vi "RGB2labMAT1.vi"(3 "sRL":dbl[](array[numeric]), 4 "sGL":dbl[](array[numeric]), 5 "sRL":dbl[](array[numeric])) -> (0 "b":dbl[](array[numeric]), 1 "a":dbl[](array[numeric]), 2 "L":dbl[](array[numeric]))   [LabVIEW 2018]
uses:
  <vilib>/Analysis/Matrix/Datatypes/RealMatrix.ctl
  <vilib>/Analysis/baseanly.llb/Real A x B.vi
  <vilib>/Analysis/NI_AALBase.lvlib
  <vilib>/Analysis/Matrix/NI_Matrix.lvlib
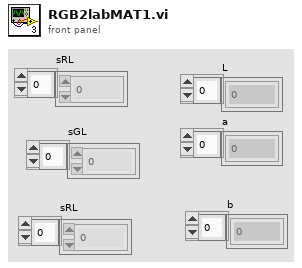
[diagram p1: front panel]
types:
  T1 = typedef "NI_Matrix.lvlib/RealMatrix.ctl" = dbl[][]
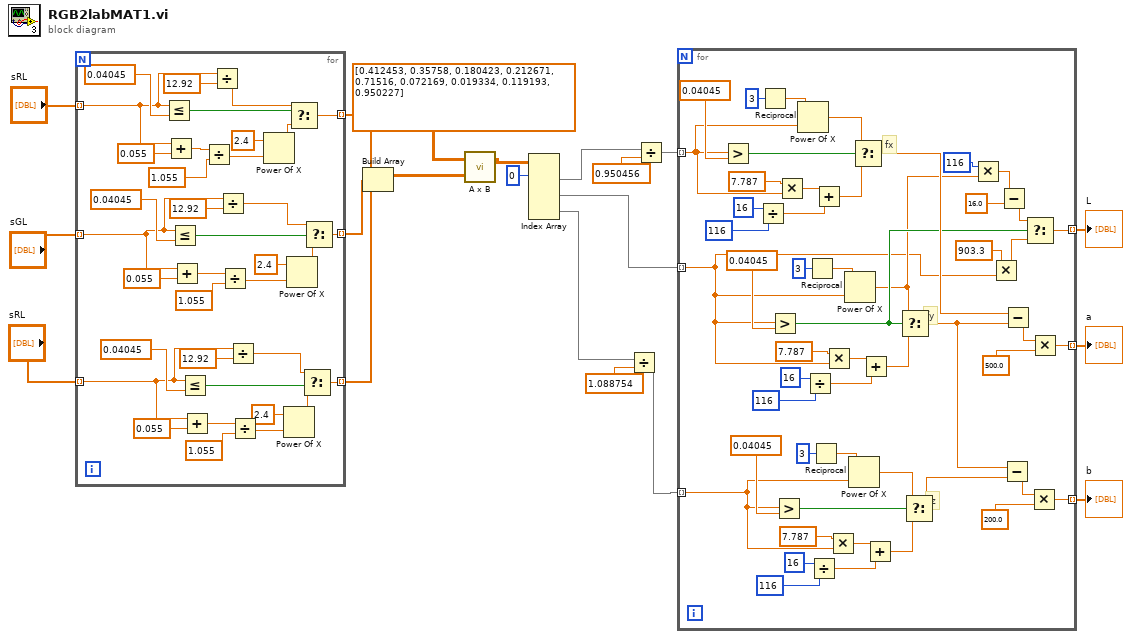
[diagram p0: block diagram]
diagram:
  n1 = for {
    tunnel: "sRL" -> [w48] mode=indexing
    tunnel: "sGL" -> [w39] mode=indexing
    tunnel: "sRL" -> [w30] mode=indexing
    tunnel: [w27] -> w17 mode=indexing
    tunnel: [w22] -> w15 mode=indexing
    tunnel: [w21] -> w16 mode=indexing
    n2 = Less Or Equal?(x=w48, y=0.04045) -> (x <= y?=w55:bool)
    n3 = Add(x=w48, y=0.055) -> (x+y=w52:dbl)
    n4 = Less Or Equal?(x=w39, y=0.04045) -> (x <= y?=w46:bool)
    n5 = Add(x=w39, y=0.055) -> (x+y=w43:dbl)
    n6 = Less Or Equal?(x=w30, y=0.04045) -> (x <= y?=w37:bool)
    n7 = Add(x=w30, y=0.055) -> (x+y=w34:dbl)
    n8 = Divide(x=w52, y=1.055) -> (x/y=w50:dbl)
    n9 = Divide(x=w48, y=12.92) -> (x/y=w29:dbl)
    n10 = Divide(x=w39, y=12.92) -> (x/y=w26:dbl)
    n11 = Divide(x=w43, y=1.055) -> (x/y=w41:dbl)
    n12 = Divide(x=w30, y=12.92) -> (x/y=w24:dbl)
    n13 = Divide(x=w34, y=1.055) -> (x/y=w32:dbl)
    n14 = Power Of X(1:w50, 2:2.4 ("y")) -> (0:w28:dbl)
    n15 = Power Of X(1:w32, 2:2.4 ("y")) -> (0:w23:dbl)
    n16 = Power Of X(1:w41, 2:2.4 ("y")) -> (0:w25:dbl)
    n17 = Select(t=w29, s=w55, f=w28) -> (s? t:f=w27:dbl)
    n18 = Select(t=w24, s=w37, f=w23) -> (s? t:f=w22:dbl)
    n19 = Select(t=w26, s=w46, f=w25) -> (s? t:f=w21:dbl)
  }
  n20 = Build Array(w17, w16, w15) -> (w14:dbl[][])
  n21 = call-poly <vilib>:"A x B.vi"("B"=w14, "A"=T1 [[0.412453, 0.35758, 0.180423], [0.212671, 0.71516, 0.072169], [0.019334, 0.119193, 0.950227]]) -> ("A x B"=w12:T1)  [unwired: 1 out]
  n22 = Index Array(array=w12, index (row) #1=0 ("索引 (行)")) -> (element #1=w10:dbl[], element #2=w5:dbl[], element #3=w7:dbl[])  [unwired: 5 in]
  n23 = Divide(x=w7, y=1.088754) -> (x/y=w4:dbl[])
  n24 = Divide(x=w10, y=0.950456) -> (x/y=w6:dbl[])
  n25 = for {
    tunnel: w6 -> [w104] mode=indexing
    tunnel: w5 -> [w59] mode=indexing
    tunnel: w4 -> [w78] mode=indexing
    tunnel: [w74] -> w2 mode=indexing
    tunnel: [w69] -> w1 mode=indexing
    tunnel: [w57] -> w3 mode=indexing
    # "fz"
    # "fy"
    # "fx"
    n26 = Greater?(x=w104, y=0.04045) -> (0:w68:bool)
    n27 = Divide(x=16, y=116) -> (x/y=w100:dbl)
    n28 = Reciprocal(x=3) -> (1/x=w106:dbl)
    n29 = Greater?(x=w59, y=0.04045) -> (0:w61:bool)
    n30 = Greater?(x=w78, y=0.04045) -> (0:w89:bool)
    n31 = Multiply(x=7.787, y=w104) -> (x*y=w103:dbl)
    n32 = Power Of X(1:w104, 2:w106) -> (0:w66:dbl)
    n33 = Divide(x=16, y=116) -> (x/y=w91:dbl)
    n34 = Reciprocal(x=3) -> (1/x=w96:dbl)
    n35 = Divide(x=16, y=116) -> (x/y=w81:dbl)
    n36 = Reciprocal(x=3) -> (1/x=w86:dbl)
    n37 = Add(x=w103, y=w100) -> (x+y=w99:dbl)
    n38 = Multiply(x=7.787, y=w59) -> (x*y=w94:dbl)
    n39 = Multiply(x=7.787, y=w78) -> (x*y=w84:dbl)
    n40 = Power Of X(1:w59, 2:w96) -> (0:w60:dbl)
    n41 = Power Of X(1:w78, 2:w86) -> (0:w79:dbl)
    n42 = Select(t=w66, s=w68, f=w99) -> (s? t:f=w77:dbl)
    n43 = Add(x=w94, y=w91) -> (x+y=w90:dbl)
    n44 = Add(x=w84, y=w81) -> (x+y=w80:dbl)
    n45 = Select(t=w60, s=w61, f=w90) -> (s? t:f=w71:dbl)
    n46 = Select(t=w79, s=w89, f=w80) -> (s? t:f=w70:dbl)
    n47 = Multiply(x=116, y=w60) -> (x*y=w64:dbl)
    n48 = Multiply(x=903.3, y=w59) -> (x*y=w58:dbl)
    n49 = Subtract(x=w64, y=16.0) -> (x-y=w65:dbl)
    n50 = Subtract(x=w71, y=w70) -> (x-y=w72:dbl)
    n51 = Subtract(x=w77, y=w71) -> (x-y=w75:dbl)
    n52 = Select(t=w65, s=w61, f=w58) -> (s? t:f=w57:dbl)
    n53 = Multiply(x=w72, y=200.0) -> (x*y=w69:dbl)
    n54 = Multiply(x=w75, y=500.0) -> (x*y=w74:dbl)
  }
  "L" <- w3
  "a" <- w2
  "b" <- w1
